vi "convert lv timestamp to unix time.vi"(11 "time stamp":timestamp) -> (3 "unix time (seconds)":dbl format="%.3f")   [LabVIEW 2013, in "Linux RT Utilities.lvlib"]
uses:
  Linux RT Utilities.lvlib
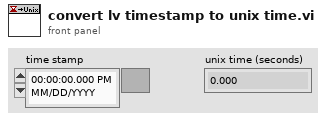
[diagram p1: front panel]
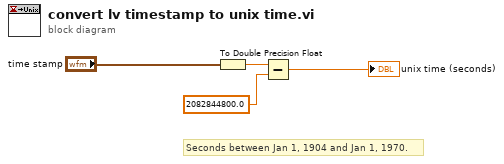
[diagram p0: block diagram]
diagram:
  # "Seconds between Jan 1, 1904 and Jan 1, 1970."
  n1 = To Double Precision Float(number="time stamp") -> (double precision float=w3:dbl)
  n2 = Subtract(x=w3, y=2082844800.0) -> (x-y=→"unix time (seconds)":dbl)
